vi "UHR-Fleezers Control (host) - 12.6.vi"() -> ()   [LabVIEW 2012] (continued)
            n2300 = Divide(x=w4104, y=w4102) -> (x/y=w4074:dbl[])
            n2301 = Divide(x=w4103, y=w4101) -> (x/y=w4073:dbl[])
            n2302 = Build Array(w4078, w4077, w4108, w4076, w4075, w4105, w4093, w4092, w4074, w4073, w4102, w4101) -> (w4097:dbl[][])
            n2303 = Bundle("T1 Y", "T1 X", "T1 Sum", "T2 Y", "T2 X", "T2 Sum", "T1 FB Sum", "T2 FB Sum", "PSD Y", "PSD X", "PSD Y Sum", "PSD X Sum") -> (w4079:T42)  [unwired: 1 out]
            n2304 = To Word Integer(number=w4112) -> (16bit integer=w4071:i16[])
            n2305 = Cluster To Array(cluster=w4079) -> (array=w4098:string[])
          }
          frame "IR-QPD + PSD + FB-QPD X position" {
            w4184 = 2  # Channel pattern
            # "time average x2 the 3 psd signals (detection laser)"
            # "deinterlace 3 signals from qpds"
            n2306 = Decimate 1D Array(w4204) -> (w4203:i16[], w4202:i16[], w4185:i16[], w4201:i16[], w4147:i16[], w4144:i16[], w4141:i16[], w4172:i16[])
            n2307 = Select(t=i16 -1, s="Flip X Sign", f=i16 1) -> (s? t:f=w4137:i16)
            n2308 = Multiply(x=w4202, y=w4137) -> (x*y=w4138:i16[])
            n2309 = Decimate 1D Array(w4185) -> (w4170:i16[], w4168:i16[])
            n2310 = Decimate 1D Array(w4203) -> (w4200:i16[], w4187:i16[])
            n2311 = Decimate 1D Array(w4138) -> (w4199:i16[], w4197:i16[])
            n2312 = Decimate 1D Array(w4201) -> (w4198:i16[], w4196:i16[])
            n2313 = Decimate 1D Array(w4172) -> (w4171:i16[], w4169:i16[])
            n2314 = call "downsample 1D array - I16.vi"("Ave N"=2.0, "Array In"=w4147) -> ("Array Out"=w4145:i16[])  [unwired: 1 in]
            n2315 = call "downsample 1D array - I16.vi"("Ave N"=2.0, "Array In"=w4141) -> ("Array Out"=w4139:i16[])  [unwired: 1 in]
            n2316 = call "downsample 1D array - I16.vi"("Ave N"=2.0, "Array In"=w4144) -> ("Array Out"=w4142:i16[])  [unwired: 1 in]
            n2317 = Interleave 1D Arrays(w4200, w4199, w4198, w4187, w4197, w4196, w4171, w4170, w4169, w4168, w4145, w4142, w4139) -> (w4195:i16[])
            n2318 = Divide(x=w4195, y=3276.7) -> (x/y=w4194:dbl[])
            n2319 = Decimate 1D Array(w4194) -> (w4193:dbl[], w4192:dbl[], w4191:dbl[], w4190:dbl[], w4189:dbl[], w4188:dbl[], w4160:dbl[], w4158:dbl[], w4157:dbl[], w4155:dbl[], w4154:dbl[], w4153:dbl[], w4150:dbl[])
            n2320 = Negate(x=w4150) -> (-x=w4148:dbl[])
            n2321 = Divide(x=w4154, y=w4150) -> (x/y=w4152:dbl[])
            n2322 = Divide(x=w4153, y=w4148) -> (x/y=w4151:dbl[])
            n2323 = Divide(x=w4193, y=w4191) -> (x/y=w4176:dbl[])
            n2324 = Divide(x=w4192, y=w4191) -> (x/y=w4175:dbl[])
            n2325 = Divide(x=w4190, y=w4188) -> (x/y=w4174:dbl[])
            n2326 = Divide(x=w4189, y=w4188) -> (x/y=w4173:dbl[])
            n2327 = Divide(x=w4160, y=w4158) -> (x/y=w4159:dbl[])
            n2328 = Divide(x=w4157, y=w4155) -> (x/y=w4156:dbl[])
            n2329 = Build Array(w4176, w4175, w4191, w4174, w4173, w4188, w4159, w4158, w4156, w4155, w4152, w4151, w4150) -> (w4149:dbl[][])
            n2330 = Bundle("T1 Y", "T1 X", "T1 Sum", "T2 Y", "T2 X", "T2 Sum", "T1 FB X", "T1 FB Sum", "T2 FB X", "T2 FB Sum", "PSD Y", "PSD X", "PSD Y Sum") -> (w4177:T43)  [unwired: 1 out]
            n2331 = Cluster To Array(cluster=w4177) -> (array=w4186:string[])
          }
          frame "IR-QPD + PSD + FB-QPD XY positions" {
            w4251 = 4  # Channel pattern
            # "time average x2 the 3 psd signals (detection laser)"
            # "deinterlace 3 signals from qpds"
            n2332 = Decimate 1D Array(w4275) -> (w4274:i16[], w4273:i16[], w4252:i16[], w4272:i16[], w4218:i16[], w4264:i16[], w4263:i16[], w4240:i16[])
            n2333 = Decimate 1D Array "Feedback Sum"(w4252) -> (w4236:i16[], w4234:i16[])
            n2334 = Decimate 1D Array "QPD Y"(w4274) -> (w4271:i16[], w4254:i16[])
            n2335 = Decimate 1D Array "QPD X"(w4273) -> (w4270:i16[], w4268:i16[])
            n2336 = Decimate 1D Array "Feedback Y"(w4218) -> (w4217:i16[], w4216:i16[])
            n2337 = Decimate 1D Array "QPD Sum"(w4272) -> (w4269:i16[], w4267:i16[])
            n2338 = Decimate 1D Array "Feedback X"(w4240) -> (w4237:i16[], w4235:i16[])
            n2339 = call "downsample 1D array - double.vi"("Ave N"=2.0, "Array In"=w4264) -> ("Array Out"=w4239:dbl[])  [unwired: 1 out]
            n2340 = call "downsample 1D array - double.vi"("Ave N"=2.0, "Array In"=w4263) -> ("Array Out"=w4238:dbl[])  [unwired: 1 out]
            n2341 = Interleave 1D Arrays(w4271, w4270, w4269, w4254, w4268, w4267, w4217, w4237, w4236, w4216, w4235, w4234, w4239, w4238) -> (w4262:dbl[])
            n2342 = Divide(x=w4262, y=3276.7) -> (x/y=w4261:dbl[])
            n2343 = Decimate 1D Array(w4261) -> (w4260:dbl[], w4259:dbl[], w4258:dbl[], w4257:dbl[], w4256:dbl[], w4255:dbl[], w4213:dbl[], w4227:dbl[], w4211:dbl[], w4212:dbl[], w4225:dbl[], w4209:dbl[], w4223:dbl[], w4221:dbl[])
            n2344 = Negate(x=w4221) -> (-x=w4219:dbl[])
            n2345 = Divide(x=w4223, y=w4219) -> (x/y=w4222:dbl[])
            n2346 = Divide(x=w4212, y=w4209) -> (x/y=w4208:dbl[])
            n2347 = Divide(x=w4213, y=w4211) -> (x/y=w4210:dbl[])
            n2348 = Divide(x=w4260, y=w4258) -> (x/y=w4244:dbl[])
            n2349 = Divide(x=w4259, y=w4258) -> (x/y=w4243:dbl[])
            n2350 = Divide(x=w4257, y=w4255) -> (x/y=w4242:dbl[])
            n2351 = Divide(x=w4256, y=w4255) -> (x/y=w4241:dbl[])
            n2352 = Divide(x=w4227, y=w4211) -> (x/y=w4226:dbl[])
            n2353 = Divide(x=w4225, y=w4209) -> (x/y=w4224:dbl[])
            n2354 = Build Array(w4244, w4243, w4258, w4242, w4241, w4255, w4210, w4226, w4211, w4208, w4224, w4209, w4222, w4221) -> (w4220:dbl[][])
            n2355 = Bundle("T1 Y", "T1 X", "T1 Sum", "T2 Y", "T2 X", "T2 Sum", "T1 FB Y", "T1 FB X", "T1 FB Sum", "T2 FB Y", "T2 FB X", "T2 FB Sum", "PSD X", "PSD Y Sum") -> (w4207:T44)  [unwired: 1 out]
            n2356 = To Word Integer(number=w4262) -> (16bit integer=w4206:i16[])
            n2357 = Cluster To Array(cluster=w4207) -> (array=w4253:string[])
          }
        }
      }
    }
    "AI labels" <- w3282
    n2358 = local read "APD Integration Time (s)"() -> (w3255:dbl)
    n2359 = Array Size(array=w3297) -> (size(s)=w3342:i32)
    n2360 = call <vilib>:"Std Deviation and Variance.vi"("X"=w3244) -> ("standard deviation"=w3243:dbl)  [unwired: 1 in, 2 out]
    n2361 = Add Array Elements(numeric array=w3244) -> (sum=w3245:u32)
    n2362 = Add Array Elements(numeric array=w3297) -> (sum=w3352:u32)
    n2363 = call <vilib>:"Std Deviation and Variance.vi"("X"=w3297) -> ("standard deviation"=w3296:dbl)  [unwired: 1 in, 2 out]
    n2364 = Divide(x=w3243, y=w3085) -> (x/y=w3240:dbl)
    "Rate sigma (Hz) 2" <- w3240
    n2365 = Multiply(x=w3085, y=w3342) -> (x*y=w3087:dbl)
    "Int. Time (s)" <- w3087
    n2366 = Divide(x=w3245, y=w3087) -> (x/y=w3241:dbl)
    "APD 2 Rate (Hz)" <- w3241
    n2367 = Multiply(x="APD Disp. Scale", y=w3248) -> (x*y=w3257:waveform(dbl)[])
    n2368 = Divide(x=w3352, y=w3087) -> (x/y=w3294:dbl)
    "APD 1 Rate (Hz)" <- w3294
    n2369 = Divide(x=w3296, y=w3085) -> (x/y=w3295:dbl)
    "Rate sigma (Hz)" <- w3295
    n2370 = Divide(x=w3240, y=w3241) -> (x/y=→"Sigma/Mean 2":dbl)
    n2371 = Multiply(x="APD Disp. Downsample", y=w3255) -> (x*y=w3253:dbl)
    n2372 = Divide(x=w3295, y=w3294) -> (x/y=→"Sigma/Mean":dbl)
    n2373 = Divide(x=w3257, y=w3253) -> (x/y=w3077:waveform(dbl)[])
    n2374 = Index Array(array=w3077, index=0) -> (element=w3237:waveform(dbl))
    n2375 = Index Array(array=w3077, index=1) -> (element=w3235:waveform(dbl))
    n2376 = Index Array(array=w3077, index=2) -> (element=w3079:waveform(dbl))
    n2377 = Subtract(x=w3237, y="APD 1 Offset") -> (x-y=w3233:waveform(dbl))
    n2378 = Subtract(x=w3235, y="APD 2 Offset") -> (x-y=w3232:waveform(dbl))
    n2379 = Subtract(x=w3079, y="APD 3 Offset") -> (x-y=w3076:waveform(dbl))
    n2380 = Add Array Elements(numeric array=w3086) -> (sum=w3089:u32)
    n2381 = call <vilib>:"Std Deviation and Variance.vi"("X"=w3086) -> ("standard deviation"=w3088:dbl)  [unwired: 1 in, 2 out]
    n2382 = Build Array(w3233, w3232, w3076) -> (→"APD Chart":waveform(dbl)[])
    n2383 = Divide(x=w3089, y=w3087) -> (x/y=w3083:dbl)
    "APD 3 Rate (Hz)" <- w3083
    n2384 = Divide(x=w3088, y=w3085) -> (x/y=w3084:dbl)
    "Rate sigma (Hz) 3" <- w3084
    n2385 = Divide(x=w3084, y=w3083) -> (x/y=→"Sigma/Mean 3":dbl)
    n2386 = local read "Data Period (s)"() -> (w3140:dbl)
    n2387 = local read "BD 1 Frequency 2 (MHz)"() -> (w3173:dbl)
    n2388 = local read "BD 1 Frequency 1 (MHz)"() -> (w3174:dbl)
    n2389 = Decimate 1D Array(w3181) -> (w3205:i16[], w3204:i16[], w3202:i16[], w3201:i16[])  [unwired: 9 out]
    n2390 = Multiply(x=w3140, y="Trap Pos. Disp. Downsample") -> (x*y=w3138:dbl)
    n2391 = Divide(x=w3205, y=w3204) -> (x/y=w3206:dbl[])
    n2392 = Divide(x=w3202, y=w3201) -> (x/y=w3203:dbl[])
    n2393 = local read "AOM X Cal (nm/MHz)"() -> (w3171:dbl)
    n2394 = Split 1D Array(array=w3206, index="N El. to Ave.") -> (second subarray=w3209:dbl[])  [unwired: 1 out]
    n2395 = Split 1D Array(array=w3203, index="N El. to Ave.") -> (second subarray=w3208:dbl[])  [unwired: 1 out]
    n2396 = Multiply(x=w3140, y="Trap Disp. Downsample") -> (x*y=w3219:dbl)
    "Display Period (s)" <- w3219
    n2397 = for "Trap AI" {
      tunnel: [w4000] -> w3384 mode=indexing
      tunnel: w3217 -> [w3991]
      tunnel: "Trap Disp. Downsample" -> [w3998]
      tunnel: w3283 -> [w3996] mode=indexing
      tunnel: w3140 -> [w3995]
      tunnel: w3282 -> [w3994] mode=indexing
      tunnel: [w3993] -> w3252 mode=indexing
      tunnel: w3219 -> [w3992]
      workers-P: _ -> [_]
      n2398 = Bundle By Name("Y"=w3996, "dt"=w3995) -> (w3997:waveform(dbl))  [unwired: 1 out]
      n2399 = Set Waveform Attribute(5:w3994, 6:"NI_ChannelName" ("name"), 7:w3997) -> (3:w3993:waveform(dbl))  [unwired: 1 in, 2 out]
      n2400 = call "downsample 1D array - double.vi"("Ave N"=w3998, "Array In"=w3996) -> ("Array Out"=w3999:dbl[])  [unwired: 1 out]
      n2401 = Bundle By Name(cluster=w3993, "t0"=w3991, "Y"=w3999, "dt"=w3992) -> (w4000:waveform(dbl))
    }
    n2402 = Bundle("BD 1 Frequency 1 (MHz)"=w3174, "BD 1 Frequency 2 (MHz)"=w3173) -> (w3175:T45)  [unwired: 1 out]
    n2403 = call-poly <vilib>:"Mean.vi"("X"=w3208) -> ("mean"=w3196:dbl)  [unwired: 1 out]
    n2404 = call-poly <vilib>:"Mean.vi"("X"=w3209) -> ("mean"=w3197:dbl)  [unwired: 1 out]
    n2405 = Reciprocal(x=w3219) -> (1/x=→"Trap Disp. Freq. (Hz)":dbl)
    n2406 = Cluster To Array(cluster=w3175) -> (array=w3172:dbl[])
    n2407 = local read "Trap X AI1 (DMA)"() -> (w3207:T13)
    n2408 = local read "Data points/scans (MCL)"() -> (w3362:dbl)
    n2409 = To Fixed-Point(number=w3196) -> (fixed-point=w3194:fxp<+/-,16,1>)  [unwired: 1 in]
    n2410 = To Fixed-Point(number=w3197) -> (fixed-point=w3195:fxp<+/-,16,1>)  [unwired: 1 in]
    n2411 = Bundle("Trap 1 Pos.", "Trap 2 Pos.") -> (w3216:cluster{string, string})  [unwired: 1 out]
    n2412 = Bundle By Name(cluster=w3207, "Set 1"=w3195, "Set 2"=w3194) -> (→"Trap X AI1 (DMA)":T13)
    n2413 = Cluster To Array(cluster=w3216) -> (array=w3213:string[])
    n2414 = Unbundle(w3073) -> (w3074:u32[])  [unwired: 2 out]
    n2415 = Select(t=-1.0, s="Negate Y Axis", f=1.0) -> (s? t:f=w3157:dbl)
    n2416 = for "Trap Position" {
      tunnel: w3221 -> [w3592] mode=indexing
      tunnel: "Trap Pos. Disp. Downsample" -> [w3591]
      tunnel: w3138 -> [w3589]
      tunnel: w3217 -> [w3588]
      tunnel: w3213 -> [w3586] mode=indexing
      tunnel: [w3585] -> w3127 mode=indexing
      tunnel: w3172 -> [w3583] mode=indexing
      tunnel: w3171 -> [w3581]
      tunnel: w3157 -> [w3580]
      n2417 = call "downsample 1D array - double.vi"("Ave N"=w3591, "Array In"=w3592) -> ("Array Out"=w3590:dbl[])  [unwired: 1 out]
      n2418 = Subtract(x=w3590, y=w3583) -> (x-y=w3584:dbl[])
      n2419 = Multiply(x=w3581, y=w3584) -> (x*y=w3582:dbl[])
      n2420 = Multiply(x=w3580, y=w3582) -> (x*y=w3579:dbl[])
      n2421 = Bundle By Name("Y"=w3579, "dt"=w3589, "t0"=w3588) -> (w3587:waveform(dbl))  [unwired: 1 out]
      n2422 = Set Waveform Attribute(5:w3586, 6:"NI_ChannelName" ("name"), 7:w3587) -> (3:w3585:waveform(dbl))  [unwired: 1 in, 2 out]
    }
    n2423 = To Double Precision Float(number=w3074) -> (double precision float=w3280:dbl[])
    n2424 = local read "Display Period (s)"() -> (w3269:dbl)
    n2425 = Increment(x=w3362) -> (x+1=w3363:dbl)
    n2426 = Index Array(array=w3127, index=0) -> (element=w3131:waveform(dbl))
    n2427 = Index Array(array=w3127, index=1) -> (element=w3126:waveform(dbl))
    n2428 = feedback #7(w3363) -> (w3366:dbl)
    n2429 = Select(t=0, s=w3353, f=w3366) -> (s? t:f=w3359:dbl)
    n2430 = Array Size(array=w3280) -> (size(s)=w3365:i32)
    n2431 = Build Array (concatenate)(w3248, w3384) -> (w3250:waveform(dbl)[])
    "All Signals" <- w3250
    n2432 = Add(x=w3365, y=w3359) -> (x+y=w3360:dbl)
    n2433 = Unbundle By Name(w3131) -> ("Y"=w3132:dbl[])
    n2434 = Divide(x="Bead Sep. Int. Time (s)", y=w3269) -> (x/y=w3167:dbl)
    n2435 = Add(x=w3132, y="FB Trap Pos Offset") -> (x+y=w3130:dbl[])
    "T1 x pos data" <- w3130
    n2436 = Greater?(x=w3360, y=w3362) -> (0:w3361:bool)
    n2437 = feedback #8(w3130) -> (w3169:dbl[])
    n2438 = Build Array (concatenate)(w3130, w3169) -> (w3168:dbl[])
    n2439 = Bundle By Name(cluster=w3131, "Y"=w3130) -> (w3129:waveform(dbl))
    n2440 = Select(t=w3359, s=w3361, f=w3360) -> (s? t:f=w3358:dbl)
    n2441 = feedback-in #7(w3358) -> ()
    n2442 = local read "MCL Scanning"() -> (w3356:bool)
    n2443 = Bundle(w3129, w3126) -> (w3125:cluster{waveform(dbl), waveform(dbl)})  [unwired: 1 out]
    n2444 = Split 1D Array(array=w3168, index=w3167) -> (first subarray=w3161:dbl[])  [unwired: 1 out]
    n2445 = feedback-in #8(w3161) -> ()
    n2446 = Not(x=w3361) -> (.not. x?=w3355:bool)
    n2447 = Cluster To Array(cluster=w3125) -> (array=w3101:waveform(dbl)[])
    "Trap Positions" <- w3101
    n2448 = call-poly <vilib>:"Mean.vi"("X"=w3161) -> ("mean"=w3160:dbl)  [unwired: 1 out]
    "Mean T1 Position (nm)" <- w3160
    n2449 = Subtract(x=w3161, y=w3160) -> (x-y=w3166:dbl[])
    n2450 = Square(x=w3166) -> (x^2=w3165:dbl[])
    n2451 = And(x=w3355, y=w3356) -> (x .and. y?=w3357:bool)
    n2452 = call-poly <vilib>:"Mean.vi"("X"=w3165) -> ("mean"=w3164:dbl)  [unwired: 1 out]
    n2453 = Square Root(x=w3164) -> (sqrt(x)=w3163:dbl)
    n2454 = Or(x=w3357, y=w3353) -> (x .or. y?=w3354:bool)
    n2455 = Equal?(x="Tab Control 6", y=T35."High Res Display") -> (x = y?=w3286:bool)
    n2456 = Multiply(x=10.0, y=w3163) -> (x*y=→"Trap 1 Position RMS (A)":dbl)
    n2457 = case "For displaying the high resolution display (no downsampling)" shown="True" w3286 {
      tunnel: w3252 -> [_ w3612]
      frame False {
      }
      frame True {
        n2458 = Index Array(array=w3612, index="High Res. Display") -> (element=w3613:waveform(dbl))
        n2459 = call <vilib>:"Std Deviation and Variance.vi"("X"=w3613) -> ("mean"=w3620:dbl, "standard deviation"=w3625:dbl)  [unwired: 1 in, 1 out]
        "Mean Intensity" <- w3620
        "Sigma" <- w3625
        n2460 = Subtract(x=w3613, y=w3620) -> (x-y=w3619:waveform(dbl))
        n2461 = Select(t=w3619, s="Subtract mean", f=w3613) -> (s? t:f=→"1 Channel":waveform(dbl))
        n2462 = Divide(x=w3625, y=w3620) -> (x/y=→"Sigma/Mean":dbl)
        n2463 = feedback #9(1) -> (w3614:i32)
        n2464 = Greater Or Equal?(x=w3614, y="Slow mean N ave.") -> (x >= y?=w3627:bool)
        n2465 = Increment(x=w3614) -> (x+1=w3629:i32)
        n2466 = Select(t=1, s=w3627, f=w3629) -> (s? t:f=w3616:i32)
        n2467 = feedback-in #9(w3616) -> ()
        n2468 = feedback #10() -> (w3617:waveform(dbl))  [unwired: 1 out]
        n2469 = case shown="Default" w3614 {
          tunnel: [w3632 w3635] -> w3618
          tunnel: w3617 -> [w3634 _]
          tunnel: w3613 -> [w3633 w3635]
          frame Default {
            n2470 = call-poly <vilib>:"Append Waveforms.vi"("waveform B"=w3633, "waveform A"=w3634) -> ("waveform out"=w3632:waveform(dbl))  [unwired: 1 in, 8 out]
          }
          frame 1 {
          }
        }
        n2471 = feedback-in #10(w3618) -> ()
        n2472 = case shown="True" w3627 {
          tunnel: w3618 -> [_ w3631]
          frame False {
          }
          frame True {
            n2473 = call-poly <vilib>:"Mean.vi"("X"=w3631) -> ("mean"=→"Slow mean":dbl)  [unwired: 1 out]
          }
        }
      }
    }
    n2474 = case "For plotting results of scanning MCL (fluorescence and detection laser images)" shown="True" w3354 {
      tunnel: w3353 -> [_ w3739]
      tunnel: w3362 -> [_ _]
      tunnel: w3252 -> [_ w3868]
      tunnel: w3230 -> [_ w3776]
      tunnel: w3073 -> [_ w3746]
      frame False {
      }
      frame True {
        w3756 = u32 0 items=["Horizontal", "Vertical", "Central", "1st Diagonal", "2nd Diagonal"] ("Type of Symmetry")
        w3783 = u32 0 items=["Horizontal", "Vertical", "Central", "1st Diagonal", "2nd Diagonal"] ("Type of Symmetry")
        w3807 = u32 0 items=["Horizontal", "Vertical", "Central", "1st Diagonal", "2nd Diagonal"] ("Type of Symmetry")
        w3810 = u32 0 items=["Horizontal", "Vertical", "Central", "1st Diagonal", "2nd Diagonal"] ("Type of Symmetry")
        w3839 = u32 0 items=["Horizontal", "Vertical", "Central", "1st Diagonal", "2nd Diagonal"] ("Type of Symmetry")
        n2475 = Unbundle(w3746) -> (w3745:u32[], w3743:u32[], w3741:u32[])
        n2476 = To Double Precision Float(number=w3745) -> (double precision float=w3744:dbl[])
        n2477 = To Double Precision Float(number=w3743) -> (double precision float=w3742:dbl[])
        n2478 = To Double Precision Float(number=w3741) -> (double precision float=w3740:dbl[])
        n2479 = Index Array(array=w3868, index=10) -> (element=w3874:waveform(dbl))
        n2480 = Index Array(array=w3868, index=11) -> (element=w3871:waveform(dbl))
        n2481 = local read "Cycles/step (MCL)"() -> (w3824:u64)
        n2482 = Index Array(array=w3868, index="Channel") -> (element=w3870:waveform(dbl))
        n2483 = Unbundle(w3776) -> ("New Image"=w3775:T2, "New Image"=w3774:T2, "New Image"=w3747:T2, "New Image"=w3748:T2, "New Image"=w3749:T2)
        n2484 = local read "Scan steps (MCL)"() -> (w3735:u64)
        n2485 = Unbundle By Name(w3874) -> ("Y"=w3826:dbl[])
        n2486 = Unbundle By Name(w3871) -> ("Y"=w3828:dbl[])
        n2487 = local read "Scan lines (y)"() -> (w3736:u64)
        n2488 = local read "N APD Samp/step"() -> (w3738:dbl)
        n2489 = Unbundle By Name(w3870) -> ("Y"=w3833:dbl[])
        n2490 = call "downsample 1D array - double.vi"("Ave N"=w3824, "Array In"=w3826) -> ("Array Out"=w3825:dbl[])  [unwired: 1 out]
        n2491 = call "downsample 1D array - double.vi"("Ave N"=w3824, "Array In"=w3828) -> ("Array Out"=w3827:dbl[])  [unwired: 1 out]
        n2492 = call "downsample 1D array - double.vi"("Ave N"=w3824, "Array In"=w3833) -> ("Array Out"=w3832:dbl[])  [unwired: 1 out]
        n2493 = Multiply(x=w3735, y=u64 2) -> (x*y=w3737:u64)
        n2494 = feedback #11(w3742) -> (w3801:dbl[])
        n2495 = Build Array (concatenate)(w3801, w3742) -> (w3800:dbl[])
        n2496 = feedback #12(w3740) -> (w3773:dbl[])
        n2497 = Build Array (concatenate)(w3773, w3740) -> (w3734:dbl[])
        n2498 = Select(t=w3742, s=w3739, f=w3800) -> (s? t:f=w3785:dbl[])
        n2499 = feedback-in #11(w3785) -> ()
        n2500 = Select(t=w3740, s=w3739, f=w3734) -> (s? t:f=w3758:dbl[])
        n2501 = feedback-in #12(w3758) -> ()
        n2502 = feedback #13(w3744) -> (w3894:dbl[])
        n2503 = Build Array (concatenate)(w3894, w3744) -> (w3876:dbl[])
        n2504 = Select(t=w3744, s=w3739, f=w3876) -> (s? t:f=w3880:dbl[])
        n2505 = feedback-in #13(w3880) -> ()
        n2506 = feedback #14(w3825) -> (w3882:dbl[])
        n2507 = Build Array (concatenate)(w3882, w3825) -> (w3873:dbl[])
        n2508 = feedback #15(w3832) -> (w3892:dbl[])
        n2509 = Build Array (concatenate)(w3892, w3832) -> (w3891:dbl[])
        n2510 = feedback #16(w3827) -> (w3884:dbl[])
        n2511 = Build Array (concatenate)(w3884, w3827) -> (w3885:dbl[])
        n2512 = Select(t=w3825, s=w3739, f=w3873) -> (s? t:f=w3829:dbl[])
        n2513 = feedback-in #14(w3829) -> ()
        n2514 = Select(t=w3832, s=w3739, f=w3891) -> (s? t:f=w3831:dbl[])
        n2515 = feedback-in #15(w3831) -> ()
        n2516 = Select(t=w3827, s=w3739, f=w3885) -> (s? t:f=w3830:dbl[])
        n2517 = feedback-in #16(w3830) -> ()
        n2518 = call "integrate 1D array interval - double.vi"("Ave N"=w3738, "Array In"=w3785) -> ("Array Out"=w3796:dbl[])  [unwired: 1 out]
        n2519 = call "integrate 1D array interval - double.vi"("Ave N"=w3738, "Array In"=w3758) -> ("Array Out"=w3769:dbl[])  [unwired: 1 out]
        n2520 = call "integrate 1D array interval - double.vi"("Ave N"=w3738, "Array In"=w3880) -> ("Array Out"=w3879:dbl[])  [unwired: 1 out]
        n2521 = Array Size(array=w3796) -> (size(s)=w3797:i32)
        n2522 = Array Size(array=w3769) -> (size(s)=w3770:i32)
        n2523 = Array Size(array=w3879) -> (size(s)=w3881:i32)
        n2524 = Multiply(x=w3736, y=w3737) -> (x*y=w3799:u64)
        n2525 = Multiply(x=w3736, y=w3737) -> (x*y=w3772:u64)
        n2526 = Multiply(x=w3736, y=w3737) -> (x*y=w3889:u64)
        n2527 = Subtract(x=w3799, y=w3797) -> (x-y=w3790:u64)
        n2528 = call-poly <vilib>:"Mean.vi"("X"=w3796) -> ("mean"=w3787:dbl)  [unwired: 1 out]
        n2529 = Subtract(x=w3772, y=w3770) -> (x-y=w3763:u64)
        n2530 = call-poly <vilib>:"Mean.vi"("X"=w3769) -> ("mean"=w3760:dbl)  [unwired: 1 out]
        n2531 = Subtract(x=w3889, y=w3881) -> (x-y=w3823:u64)
        n2532 = call-poly <vilib>:"Mean.vi"("X"=w3879) -> ("mean"=w3820:dbl)  [unwired: 1 out]
        n2533 = call-poly <vilib>:"Mean.vi"("X"=w3829) -> ("mean"=w3813:dbl)  [unwired: 1 out]
        n2534 = call-poly <vilib>:"Mean.vi"("X"=w3831) -> ("mean"=w3818:dbl)  [unwired: 1 out]
        n2535 = call-poly <vilib>:"Mean.vi"("X"=w3830) -> ("mean"=w3816:dbl)  [unwired: 1 out]
        n2536 = Initialize Array(1.0 ("element"), w3790) -> (w3786:dbl[])
        n2537 = Initialize Array(1.0 ("element"), w3763) -> (w3759:dbl[])
        n2538 = Initialize Array(1.0 ("element"), w3823) -> (w3814:dbl[])
        n2539 = Multiply(x=w3786, y=w3787) -> (x*y=w3788:dbl[])
        n2540 = Multiply(x=w3759, y=w3760) -> (x*y=w3761:dbl[])
        n2541 = Multiply(x=w3814, y=w3820) -> (x*y=w3821:dbl[])
        n2542 = Multiply(x=w3814, y=w3816) -> (x*y=w3817:dbl[])
        n2543 = Multiply(x=w3814, y=w3818) -> (x*y=w3819:dbl[])
        n2544 = Multiply(x=w3814, y=w3813) -> (x*y=w3815:dbl[])
        n2545 = Build Array (concatenate)(w3796, w3788) -> (w3798:dbl[])
        n2546 = Build Array (concatenate)(w3769, w3761) -> (w3771:dbl[])
        n2547 = Build Array (concatenate)(w3879, w3821) -> (w3888:dbl[])
        n2548 = Build Array (concatenate)(w3829, w3815) -> (w3883:dbl[])
        n2549 = Build Array (concatenate)(w3831, w3819) -> (w3887:dbl[])
        n2550 = Build Array (concatenate)(w3830, w3817) -> (w3886:dbl[])
        n2551 = Reshape Array(w3798, w3736, w3737) -> (w3794:dbl[][])
        n2552 = Reshape Array(w3771, w3736, w3737) -> (w3767:dbl[][])
        n2553 = Reshape Array(w3888, w3736, w3737) -> (w3866:dbl[][])
        n2554 = Reshape Array(w3883, w3736, w3737) -> (w3849:dbl[][])
        n2555 = Reshape Array(w3887, w3736, w3737) -> (w3841:dbl[][])
        n2556 = Reshape Array(w3886, w3736, w3737) -> (w3856:dbl[][])
        n2557 = Array Subset(array=w3794, index (col)=0 ("index"), length (col)=w3735) -> (w3793:dbl[][])  [unwired: 2 in]
        n2558 = Array Subset(array=w3794, index (col)=w3735) -> (w3791:dbl[][])  [unwired: 3 in]
        n2559 = Array Subset(array=w3767, index (col)=0 ("index"), length (col)=w3735) -> (w3766:dbl[][])  [unwired: 2 in]
        n2560 = Array Subset(array=w3767, index (col)=w3735) -> (w3764:dbl[][])  [unwired: 3 in]
        n2561 = Array Subset(array=w3856, index (col)=0 ("index"), length (col)=w3735) -> (w3861:dbl[][])  [unwired: 2 in]
        n2562 = Array Subset(array=w3856, index (col)=w3735) -> (w3859:dbl[][])  [unwired: 3 in]
        n2563 = Array Subset(array=w3866, index (col)=0 ("index"), length (col)=w3735) -> (w3865:dbl[][])  [unwired: 2 in]
        n2564 = Array Subset(array=w3866, index (col)=w3735) -> (w3863:dbl[][])  [unwired: 3 in]
        n2565 = Array Subset(array=w3841, index (col)=0 ("index"), length (col)=w3735) -> (w3847:dbl[][])  [unwired: 2 in]
        n2566 = Array Subset(array=w3841, index (col)=w3735) -> (w3845:dbl[][])  [unwired: 3 in]
        n2567 = Array Subset(array=w3849, index (col)=0 ("index"), length (col)=w3735) -> (w3854:dbl[][])  [unwired: 2 in]
        n2568 = Array Subset(array=w3849, index (col)=w3735) -> (w3852:dbl[][])  [unwired: 3 in]
        n2569 = for {
          tunnel: w3793 -> [w3898] mode=indexing
          tunnel: [w3897] -> w3792 mode=indexing
          workers-P: _ -> [_]
          n2570 = Reverse 1D Array(array=w3898) -> (reversed array=w3897:dbl[])
        }
        n2571 = for {
          tunnel: w3766 -> [w3896] mode=indexing
          tunnel: [w3895] -> w3765 mode=indexing
          workers-P: _ -> [_]
          n2572 = Reverse 1D Array(array=w3896) -> (reversed array=w3895:dbl[])
        }
        n2573 = for {
          tunnel: w3861 -> [w3904] mode=indexing
          tunnel: [w3903] -> w3860 mode=indexing
          workers-P: _ -> [_]
          n2574 = Reverse 1D Array(array=w3904) -> (reversed array=w3903:dbl[])
        }
        n2575 = for {
          tunnel: w3865 -> [w3906] mode=indexing
          tunnel: [w3905] -> w3864 mode=indexing
          workers-P: _ -> [_]
          n2576 = Reverse 1D Array(array=w3906) -> (reversed array=w3905:dbl[])
        }
        n2577 = for {
          tunnel: w3847 -> [w3900] mode=indexing
          tunnel: [w3899] -> w3846 mode=indexing
          workers-P: _ -> [_]
          n2578 = Reverse 1D Array(array=w3900) -> (reversed array=w3899:dbl[])
        }
        n2579 = for {
          tunnel: w3854 -> [w3902] mode=indexing
          tunnel: [w3901] -> w3853 mode=indexing
          workers-P: _ -> [_]
          n2580 = Reverse 1D Array(array=w3902) -> (reversed array=w3901:dbl[])
        }
        n2581 = Index Array(array=w3866, index (row)=0) -> (element=→"Waveform Graph":dbl[])  [unwired: 1 in]
        n2582 = Add(x=w3792, y=w3791) -> (x+y=w3778:dbl[][])
        n2583 = Add(x=w3765, y=w3764) -> (x+y=w3751:dbl[][])
        n2584 = Add(x=w3860, y=w3859) -> (x+y=w3858:dbl[][])
        n2585 = Add(x=w3864, y=w3863) -> (x+y=w3838:dbl[][])
        n2586 = Add(x=w3846, y=w3845) -> (x+y=w3844:dbl[][])
        n2587 = Add(x=w3853, y=w3852) -> (x+y=w3851:dbl[][])
        n2588 = Divide(x=w3844, y=2) -> (x/y=w3842:dbl[][])
        n2589 = Divide(x=w3858, y=2) -> (x/y=w3803:dbl[][])
        n2590 = To Single Precision Float(number=w3838) -> (single precision float=w3837:sgl[][])
        n2591 = To Single Precision Float(number=w3778) -> (single precision float=w3782:sgl[][])
        n2592 = To Single Precision Float(number=w3751) -> (single precision float=w3755:sgl[][])
        n2593 = Divide(x=w3851, y=2) -> (x/y=w3805:dbl[][])
        n2594 = Transpose 2D Array(2D array=w3842) -> (transposed array=→"Data map":dbl[][])
        n2595 = To Single Precision Float(number=w3803) -> (single precision float=w3809:sgl[][])
        n2596 = To Single Precision Float(number=w3805) -> (single precision float=w3806:sgl[][])
        n2597 = call "IMAQ ArrayToImage"("Image Pixels (Float)"=w3837, "Image"=w3775) -> ("Image Out"=w3840:T2)  [unwired: 8 in, 1 out]
        n2598 = call "IMAQ ArrayToImage"("Image Pixels (Float)"=w3782, "Image"=w3774) -> ("Image Out"=w3784:T2)  [unwired: 8 in, 1 out]
        n2599 = call "IMAQ ArrayToImage"("Image Pixels (Float)"=w3755, "Image"=w3747) -> ("Image Out"=w3757:T2)  [unwired: 8 in, 1 out]
        n2600 = call "IMAQ ArrayToImage"("Image Pixels (Float)"=w3809, "Image"=w3748) -> ("Image Out"=w3811:T2)  [unwired: 8 in, 1 out]
        n2601 = call "IMAQ Symmetry"("Type of Symmetry"=w3839, "Image Src"=w3840) -> ("Image Dst Out"=w3835:T2)  [unwired: 3 in, 1 out]
        n2602 = call "IMAQ ArrayToImage"("Image Pixels (Float)"=w3806, "Image"=w3749) -> ("Image Out"=w3808:T2)  [unwired: 8 in, 1 out]
        n2603 = call "IMAQ Symmetry"("Type of Symmetry"=w3783, "Image Src"=w3784) -> ("Image Dst Out"=w3780:T2)  [unwired: 3 in, 1 out]
        n2604 = call "IMAQ Symmetry"("Type of Symmetry"=w3756, "Image Src"=w3757) -> ("Image Dst Out"=w3753:T2)  [unwired: 3 in, 1 out]
        n2605 = call "IMAQ Symmetry"("Type of Symmetry"=w3810, "Image Src"=w3811) -> ("Image Dst Out"=→"Detection Laser X":T2)  [unwired: 3 in, 1 out]
        n2606 = call "IMAQ Symmetry"("Type of Symmetry"=w3807, "Image Src"=w3808) -> ("Image Dst Out"=→"Detection Laser Y":T2)  [unwired: 3 in, 1 out]
        n2607 = call "IMAQ Set Simple Calibration"("Calibration Axis Info"=T36 {"Origin Pixel"={"X"=0.0, "Y"=0.0}, "Angle Relative to Horizontal (deg)"=0.0, "Axis Reference"=0}, "Grid Descriptor"=T37 {"X Step"=0.3, "Y Step"=0.3, "Unit"=enum."Undefined"}, "Image"=w3835) -> ("Calibrated Image"=→"APD 1":T2)  [unwired: 7 in, 1 out]
        n2608 = call "IMAQ Set Simple Calibration"("Calibration Axis Info"=T36 {"Origin Pixel"={"X"=0.0, "Y"=0.0}, "Angle Relative to Horizontal (deg)"=0.0, "Axis Reference"=0}, "Grid Descriptor"=T37 {"X Step"=0.3, "Y Step"=0.3, "Unit"=enum."Undefined"}, "Image"=w3780) -> ("Calibrated Image"=→"APD 2":T2)  [unwired: 7 in, 1 out]
        n2609 = call "IMAQ Set Simple Calibration"("Calibration Axis Info"=T36 {"Origin Pixel"={"X"=0.0, "Y"=0.0}, "Angle Relative to Horizontal (deg)"=0.0, "Axis Reference"=0}, "Grid Descriptor"=T37 {"X Step"=0.3, "Y Step"=0.3, "Unit"=enum."Undefined"}, "Image"=w3753) -> ("Calibrated Image"=→"APD 3":T2)  [unwired: 7 in, 1 out]
      }
    }
    n2610 = case "For computing FFTs for display" shown="True" "Compute FFT" {
      tunnel: w3252 -> [_ w4378]
      frame False {
      }
      frame True {
        n2611 = Build Array("FFT 1 Choice 1", "FFT 1 Choice 2", "FFT 2 Choice 1", "FFT 2 Choice 2") -> (w4371:u16[])
        n2612 = Array Size(array=w4378) -> (size(s)=w4377:i32)
        n2613 = feedback-in #17(w4371) -> ()
        n2614 = feedback #17(u16[] [100, 100, 100, 100]) -> (w4372:u16[])
        n2615 = feedback-in #18("# Spectra to Ave.") -> ()
        n2616 = feedback #18("# Spectra to Ave.") -> (w4369:dbl)
        n2617 = Not Equal?(x="# Spectra to Ave.", y=w4369) -> (x != y?=w4368:bool)
        n2618 = Not Equal?(x=w4371, y=w4372) -> (x != y?=w4370:bool)
        n2619 = feedback #19(1.0) -> (w4355:dbl)
        n2620 = Compound Arithmetic op=OR("Reset FFT", w4370, w4368) -> (w4353:bool)
        n2621 = Select(t=1.0, s=w4353, f=w4355) -> (s? t:f=w4357:dbl)
        n2622 = Greater?(x=w4357, y="# Spectra to Ave.") -> (0:w4376:bool)
        n2623 = Increment(x=w4357) -> (x+1=w4356:dbl)
        n2624 = feedback-in #19(w4356) -> ()
        n2625 = local read "DMA Update Period (s)"() -> (w4351:dbl)
        n2626 = Multiply(x="# Spectra to Ave.", y=w4351) -> (x*y=→"Ave. Time (s)":dbl)
        n2627 = Build Array(cluster{"f0":dbl, "df":dbl, "magnitude":dbl[]} {"f0"=0.0, "df"=0.0, "magnitude"=[]} ("PSD")) -> (w4360:cluster{"f0":dbl, "df":dbl, "magnitude":dbl[]}[])
        n2628 = Build Array(w4360, w4360, w4360, w4360) -> (w4362:T46)
        n2629 = feedback #20(w4362) -> (w4367:T46)
        n2630 = for {
          N: 4 -> [_]
          tunnel: w4371 -> [w4400] mode=indexing
          tunnel: w4378 -> [w4401]
          tunnel: w4377 -> [w4403]
          tunnel: w4353 -> [w4396]
          tunnel: w4376 -> [w4395]
          tunnel: "# Spectra to Ave." -> [w4394]
          tunnel: [w4393] -> w4366 mode=indexing
          tunnel: w4367 -> [w4398] mode=indexing
          tunnel: [w4397] -> w4354 mode=indexing
          tunnel: w4357 -> [w4392]
          n2631 = Less?(x=w4400, y=w4403) -> (x < y?=w4402:bool)
          n2632 = Index Array(array=w4401, index=w4400) -> (element=w4399:waveform(dbl))
          n2633 = case shown="True" w4402 {
            tunnel: w4399 -> [_ w4420]
            tunnel: w4398 -> [w4405 w4418]
            tunnel: [w4405 w4406] -> w4397
            tunnel: w4396 -> [_ w4417]
            tunnel: w4395 -> [_ w4410]
            tunnel: w4394 -> [_ w4409]
            tunnel: [cluster{"f0":dbl, "df":dbl, "magnitude":dbl[]} {"f0"=0.0, "df"=0.0, "magnitude"=[]} ("PSD") w4411] -> w4393
            tunnel: w4392 -> [_ w4408]
            frame False {
            }
            frame True {
              n2634 = call <vilib>:"Std Deviation and Variance.vi"("X"=w4420) -> ("mean"=w4421:dbl)  [unwired: 1 in, 2 out]
              n2635 = Subtract(x=w4420, y=w4421) -> (x-y=w4419:waveform(dbl))
              n2636 = xnode "Spectral Measurements"("Signals"=w4419) -> ("PSD"=w4413:cluster{"f0":dbl, "df":dbl, "magnitude":dbl[]})  [unwired: 1 in, 1 out]
              n2637 = case shown="False" w4417 {
                tunnel: w4418 -> [w4430 _]
                tunnel: [w4426 w4435] -> w4406
                tunnel: w4413 -> [w4429 w4436]
                tunnel: w4410 -> [w4428 _]
                frame False {
                  n2638 = Build Array (concatenate)(w4430, w4429) -> (w4427:cluster{"f0":dbl, "df":dbl, "magnitude":dbl[]}[])
                  n2639 = case shown="True" w4428 {
                    tunnel: w4427 -> [w4431 w4434]
                    tunnel: [w4431 w4432] -> w4426
                    frame False {
                    }
                    frame True {
                      n2640 = Delete From Array(array=w4434, index=0) -> (array with subset deleted=w4432:cluster{"f0":dbl, "df":dbl, "magnitude":dbl[]}[])  [unwired: 1 in, 1 out]
                    }
                  }
                }
                frame True {
                  n2641 = Build Array(w4436) -> (w4435:cluster{"f0":dbl, "df":dbl, "magnitude":dbl[]}[])
                }
              }
              n2642 = for {
                tunnel: w4406 -> [w4425] mode=indexing
                tunnel: [w4424] -> w4416 mode=indexing
                workers-P: _ -> [_]
                n2643 = Unbundle By Name(w4425) -> ("magnitude"=w4424:dbl[])
              }
              n2644 = Transpose 2D Array(2D array=w4416) -> (transposed array=w4415:dbl[][])
              n2645 = for {
                tunnel: w4415 -> [w4423] mode=indexing
                tunnel: [w4422] -> w4414 mode=indexing
                workers-P: _ -> [_]
                n2646 = Add Array Elements(numeric array=w4423) -> (sum=w4422:dbl)
              }
              n2647 = Select(t=w4409, s=w4410, f=w4408) -> (s? t:f=w4407:dbl)
              n2648 = Divide(x=w4414, y=w4407) -> (x/y=w4412:dbl[])
              n2649 = Bundle By Name(cluster=w4413, "magnitude"=w4412) -> (w4411:cluster{"f0":dbl, "df":dbl, "magnitude":dbl[]})
            }
          }
        }
        n2650 = case shown="True" w4353 {
          tunnel: w4354 -> [w4385 w4391]
          tunnel: [w4385 w4386] -> w4352
          frame False {
          }
          frame True {
            n2651 = Array Subset(array=w4391, index (row)=0 ("index"), length (row)=4 ("length"), index (col)=0 ("index"), length (col)=1 ("length")) -> (w4386:T46)
          }
        }
        n2652 = feedback-in #20(w4352) -> ()
        n2653 = Split 1D Array(array=w4366, index=2) -> (first subarray=→"FFT 1":cluster{"f0":dbl, "df":dbl, "magnitude":dbl[]}[], second subarray=→"FFT 2":cluster{"f0":dbl, "df":dbl, "magnitude":dbl[]}[])
      }
    }
    n2654 = Index Array(array=w3250, index=4) -> (element=w3306:waveform(dbl))
    n2655 = Index Array(array=w3250, index=7) -> (element=w3303:waveform(dbl))
    n2656 = Divide(x="T1 offset_x (mV)", y=1000.0) -> (x/y=w3307:dbl)
    n2657 = feedback-in #21("Calibration") -> ()
    n2658 = feedback #21(u16 1 ("Calibration")) -> (w3325:u16)
    n2659 = Divide(x="T2 offset_x (mV)", y=1000.0) -> (x/y=w3305:dbl)
    n2660 = case shown="2" "Calibration" {
      tunnel: "T1 alpha_x (nm/V)" -> [_ w3699 w3720]
      tunnel: "T1 kappa_x (pN/nm)" -> [_ _ w3710]
      tunnel: "T2 alpha_x (nm/V)" -> [_ w3698 w3718]
      tunnel: "T2 kappa_x (pN/nm)" -> [_ _ w3711]
      tunnel: w3306 -> [w3681 w3696 w3716]
      tunnel: w3303 -> [w3680 w3694 w3714]
      tunnel: [w3681 w3693 w3713] -> w3334
      tunnel: [w3680 w3692 w3712] -> w3333
      tunnel: ["T1 X (V)" ("Label.Text") "T1 X (nm)" ("Label.Text") "T1 X (pN)" ("Label.Text")] -> w3322
      tunnel: ["T2 X (V)" ("Label.Text") "T2 X (nm)" ("Label.Text") "T2 X (pN)" ("Label.Text")] -> w3321
      tunnel: ["Position (V)" ("Label.Text") "Position (nm)" ("Label.Text") "Force (pN)" ("Label.Text")] -> w3323
      tunnel: w3305 -> [_ w3684 w3703]
      tunnel: w3307 -> [_ w3687 w3705]
      tunnel: ["Mean (V)" ("Label.Text") "Mean (nm)" ("Label.Text") "Mean (pN)" ("Label.Text")] -> w3318
      tunnel: ["Difference (V)" ("Label.Text") "Difference (nm)" ("Label.Text") "Difference (pN)" ("Label.Text")] -> w3258
      frame 0, Default {
      }
      frame 1 {
        n2661 = Unbundle By Name(w3696) -> ("Y"=w3700:dbl[])
        n2662 = Unbundle By Name(w3694) -> ("Y"=w3685:dbl[])
        n2663 = Subtract(x=w3700, y=w3687) -> (x-y=w3688:dbl[])
        n2664 = Subtract(x=w3685, y=w3684) -> (x-y=w3686:dbl[])
        n2665 = Multiply(x=w3686, y=w3698) -> (x*y=w3695:dbl[])
        n2666 = Multiply(x=w3699, y=w3688) -> (x*y=w3697:dbl[])
        n2667 = Bundle By Name(cluster=w3694, "Y"=w3695) -> (w3692:waveform(dbl))
        n2668 = Bundle By Name(cluster=w3696, "Y"=w3697) -> (w3693:waveform(dbl))
      }
      frame 2 {
        n2669 = Unbundle By Name(w3716) -> ("Y"=w3721:dbl[])
        n2670 = Unbundle By Name(w3714) -> ("Y"=w3719:dbl[])
        n2671 = Subtract(x=w3719, y=w3703) -> (x-y=w3704:dbl[])
        n2672 = Subtract(x=w3721, y=w3705) -> (x-y=w3706:dbl[])
        n2673 = Compound Arithmetic op=MULTIPLY(w3704, w3718, w3711) -> (w3715:dbl[])
        n2674 = Compound Arithmetic op=MULTIPLY(w3710, w3720, w3706) -> (w3717:dbl[])
        n2675 = Bundle By Name(cluster=w3714, "Y"=w3715) -> (w3712:waveform(dbl))
        n2676 = Bundle By Name(cluster=w3716, "Y"=w3717) -> (w3713:waveform(dbl))
      }
    }
    n2677 = case shown="True" "Read Lateness and Rel Phase" {
      tunnel: w3124 -> [w3636 w3669]
      tunnel: w3123 -> [w3637 w3668]
      tunnel: [w3636 w3641] -> w3300
      tunnel: [w3637 w3640] -> w3299
      frame False {
      }
      frame True {
        n2678 = xnode "Read/Write Control"("FPGA VI Reference In"=w3669, "error in"=w3668) -> ("FPGA VI Reference Out"=w3643:T20, "error out"=w3642:errorcluster, "GI Relative phase"=→"GI relative phase":i16, "Relative phase"=→"Relative phase (AI1)":i16, "AI Late Counter"=→"Late Counter (AI1)":u8, "GI Late Counter"=→"GI Late Counter":u8, "MCL Late Counter"=→"MCL Late Counter":u8, "MCL Relative Phase"=→"Relative Phase (MCL)":i16, "APD Acq Relative Phase"=→"APD Acq Relative Phase":i16, "APD 1 Gate Relative Phase"=→"APD 1 Gate Relative Phase":i16, "APD 2 Gate Relative Phase"=→"APD 2 Gate Relative Phase":i16, "APD Acq Late Counter"=→"APD Acq Late Counter":u8, "APD 1 Gate Late Counter"=→"APD 1 Gate Late Counter":u8, "APD 2 Gate Late Counter"=→"APD 2 Gate Late Counter":u8, "Green FB Relative Phase"=→"Relative phase (Green FB)":i16, "GI Relative phase 2"=→"GI relative phase 2":i16, "GI Late Counter 2"=→"GI Late Counter 2":u8, "Trap Pos FIFO Timeout"=→"Trap Pos FIFO Timeout":u16, "Trap AI FIFO Timeout"=→"Trap AI FIFO Timeout":u16, "RI Late Counter"=→"RI Late Counter":u8, "RI Relative phase"=→"RI relative phase":i16, "Green Late Counter"=→"Green AI Late Counter":u8, "BI Late Counter (AO)"=→"Late Counter (BI AO)":u8, "Blue Late Counter (D)"=→"Late Counter (BI DO)":u8, "BI Relative phase (AO)"=→"Relative phase (BI AO)":i16, "BI Relative phase (D)"=→"Relative phase (BI DO)":i16)
        n2679 = xnode "Read/Write Control"("FPGA VI Reference In"=w3643, "error in"=w3642) -> ("FPGA VI Reference Out"=w3641:T20, "error out"=w3640:errorcluster, "APD 3 Gate Late Counter"=→"APD 3 Gate Late Counter":u8, "APD 3 Gate Relative Phase"=→"APD 3 Gate Relative Phase":i16)
      }
    }
    n2680 = Not Equal?(x=w3325, y="Calibration") -> (x != y?=w3284:bool)
    n2681 = case shown="True" w3284 {
      tunnel: w3323 -> [_ w3674]
      tunnel: w3322 -> [_ w3673]
      tunnel: w3321 -> [_ w3672]
      tunnel: w3318 -> [_ w3671]
      tunnel: w3258 -> [_ w3670]
      frame False {
      }
      frame True {
        n2682 = property on="Force" class="WFChart (strict)"("YScale.NameLbl.Text"=w3674) -> ()  [unwired: 2 in, 2 out]
        n2683 = property on="T2 X" class="DigNum (strict)"("Caption.Text"=w3672) -> ()  [unwired: 2 in, 2 out]
        n2684 = property on="T1 X" class="DigNum (strict)"("Caption.Text"=w3673) -> ()  [unwired: 2 in, 2 out]
        n2685 = property on="Mean" class="DigNum (strict)"("Caption.Text"=w3671) -> ()  [unwired: 2 in, 2 out]
        n2686 = property on="Difference" class="DigNum (strict)"("Caption.Text"=w3670) -> ()  [unwired: 2 in, 2 out]
      }
    }
    n2687 = Unbundle By Name(w3306) -> ("Y"=w3309:dbl[])
    n2688 = Unbundle By Name(w3303) -> ("Y"=w3312:dbl[])
    n2689 = Subtract(x=w3309, y=w3307) -> (x-y=w3310:dbl[])
    n2690 = Subtract(x=w3312, y=w3305) -> (x-y=w3311:dbl[])
    n2691 = Multiply(x=w3311, y="T2 alpha_x (nm/V)") -> (x*y=w3106:dbl[])
    n2692 = Multiply(x="T1 alpha_x (nm/V)", y=w3310) -> (x*y=w3107:dbl[])
    n2693 = Not(x="Trap Trig. Fl.") -> (.not. x?=w3143:bool)
    n2694 = Multiply(x=w3333, y=-1.0) -> (x*y=w3314:waveform(dbl))
    n2695 = Subtract(x=w3107, y=w3106) -> (x-y=w3302:dbl[])
    n2696 = Unbundle By Name(w3333) -> ("Y"=w3274:dbl[])
    n2697 = Unbundle By Name(w3334) -> ("Y"=w3108:dbl[])
    n2698 = Negate(x=w3302) -> (-x=w3104:dbl[])
    n2699 = Build Array(w3334, w3314) -> (→"Force":waveform(dbl)[])
    n2700 = Subtract(x=w3104, y="Offset (nm)") -> (x-y=w3272:dbl[])
    n2701 = call-poly <vilib>:"Mean.vi"("X"=w3274) -> ("mean"=w3110:dbl)  [unwired: 1 out]
    "T2 X" <- w3110
    n2702 = Negate(x=w3274) -> (-x=w3275:dbl[])
    n2703 = call-poly <vilib>:"Mean.vi"("X"=w3108) -> ("mean"=w3111:dbl)  [unwired: 1 out]
    "T1 X" <- w3111
    n2704 = Negate(x=w3110) -> (-x=w3109:dbl)
    n2705 = Bundle By Name(cluster=w3306, "Y"=w3272) -> (w3249:waveform(dbl))
    "Bead Separation" <- w3249
    n2706 = Add(x=w3108, y=w3275) -> (x+y=w3276:dbl[])
    n2707 = Add(x=w3111, y=w3109) -> (x+y=w3320:dbl)
    n2708 = Subtract(x=w3111, y=w3109) -> (x-y=→"Difference":dbl)
    n2709 = Divide(x=w3276, y=2.0) -> (x/y=→"Vec Mean of T1 T2":dbl[])
    n2710 = Divide(x=w3320, y=2.0) -> (x/y=w3278:dbl)
    "Mean" <- w3278
    n2711 = feedback-in #22("Trap Trig. Fl.") -> ()
    n2712 = feedback #22("Trap Trig. Fl.") -> (w3141:bool)
    n2713 = And(x=w3143, y=w3141) -> (x .and. y?=w3142:bool)
    n2714 = case "If have just turned off triggering" shown="True" w3142 {
      tunnel: w3124 -> [_ w3471]
      tunnel: w3123 -> [_ w3470]
      frame False {
      }
      frame True {
        w3469 = FALSE ("FPGA Trap Trig")
        n2715 = xnode "Read/Write Control"("FPGA VI Reference In"=w3471, "error in"=w3470, "FPGA Trap Trig"=w3469) -> ("FPGA VI Reference Out"=w3468:T20, "error out"=w3467:errorcluster)
        n2716 = xnode "Read/Write Control"("FPGA VI Reference In"=w3468, "error in"=w3467, "TTrig?"=w3469) -> ()  [unwired: 2 out]
        n2717 = local write "Initializing"(FALSE ("Initializing")) -> ()
        n2718 = local write "Triggered"(FALSE ("Triggered")) -> ()
        n2719 = local write "Waiting"(FALSE ("Waiting")) -> ()
      }
    }
    n2720 = Not(x=w3141) -> (.not. x?=w3154:bool)
    n2721 = And(x="Trap Trig. Fl.", y=w3154) -> (x .and. y?=w3151:bool)
    n2722 = local read "Tether"() -> (w3279:bool)
    n2723 = Or(x=w3151, y="Reinitialize") -> (x .or. y?=w3137:bool)
    n2724 = feedback #23(w3147) -> (w3152:string)
    n2725 = Select(t=w3147, s=w3151, f=w3152) -> (s? t:f=w3146:string)
    n2726 = Select(t=w3147, s="Reinitialize", f=w3146) -> (s? t:f=w3145:string)
    n2727 = feedback #24(0) -> (w3149:i32)
    n2728 = feedback #25(w3272) -> (w3271:dbl[])
    n2729 = Build Array (concatenate)(w3272, w3271) -> (w3105:dbl[])
    n2730 = case "For determining if there is a tether still" shown="True" w3279 {
      tunnel: w3278 -> [_ w3595]
      frame False {
      }
      frame True {
        n2731 = Greater?(x="Lost Tether Alarm Threshold (pN)", y=w3595) -> (0:w3593:bool)
        n2732 = case shown="True" w3593 {
          frame False {
          }
          frame True {
            w3596 = FALSE ("Value (Signaling)")
            n2733 = flat-sequence {
              frame #0 {
                # "stop only if saving"
                n2734 = local read "Saving..."() -> (w3608:bool)
                n2735 = And(x=w3608, y="TA Cancel Save?") -> (x .and. y?=w3607:bool)
                n2736 = local write "Stop Saving"(w3607) -> ()
              }
              frame #1 {
                n2737 = case shown="True" "TA Green Off?" {
                  frame False {
                  }
                  frame True {
                    w3611 = FALSE ("Fl. Triggered...")
                    n2738 = local write "Fl. Triggered..."(w3611) -> ()
                    n2739 = property on="Green Laser ON" class="Bool (strict)"("Val(Sgnl)"=w3611) -> ()  [unwired: 2 in, 2 out]
                  }
                }
              }
            }
            n2740 = local read "Time tether formed"() -> (w3602:timestamp)
            n2741 = Get Date/Time In Seconds() -> (seconds since 1Jan1904=w3603:timestamp)
            n2742 = Subtract(x=w3603, y=w3602) -> (x-y=w3601:dbl)
            n2743 = Number To Decimal String(number=w3601) -> (decimal integer string=w3598:string)  [unwired: 1 out]
            n2744 = local read "Messages"() -> (w3605:string)
            n2745 = call <vilib>:"Beep.vi"() -> ()  [unwired: 3 in, 9 out]
            n2746 = Concatenate Strings("Lost tether (" ("Message to add"), w3598, " s)." ("string")) -> (w3600:string)
            n2747 = local write "Tether"(FALSE ("Tether")) -> ()
            n2748 = call "Update messages.vi"("Message to add"=w3600, "Old message string"=w3605) -> ("New message string"=w3604:string)
            n2749 = local write "Messages"(w3604) -> ()
            n2750 = property on="Fl. Triggered..." class="Bool (strict)"("Val(Sgnl)"=w3596) -> ()  [unwired: 2 in, 2 out]
            n2751 = local write "Dip for Protein"(w3596) -> ()
            n2752 = property on="Trap Pos. FB ON" class="Bool (strict)"("Val(Sgnl)"=w3596) -> ()  [unwired: 2 in, 2 out]
            n2753 = property on="Trap Trig. Fl." class="Bool (strict)"("Val(Sgnl)"=w3596) -> ()  [unwired: 2 in, 2 out]
          }
        }
      }
    }
    n2754 = case "For triggering actions based on the trap position (e.g., turning the excitation laser on if trap under feedback moves so far)" shown="True" "Trap Trig. Fl." {
      tunnel: w3132 -> [_ w3484]
      tunnel: w3145 -> [_ w3483]
      tunnel: ["" ("t") w3482] -> w3153
      tunnel: w3137 -> [_ w3481]
      tunnel: [0 ("t") w3480] -> w3150
      tunnel: w3149 -> [_ w3479]
      tunnel: w3124 -> [_ w3478]
      tunnel: w3123 -> [_ w3477]
      frame False {
      }
      frame True {
        n2755 = case shown="\"Wait for trigger\"" w3483 {
          tunnel: w3484 -> [w3501 _ _ w3549]
          tunnel: [w3498 w3530 "" ("t") w3552] -> w3482
          tunnel: w3481 -> [_ _ _ w3540]
          tunnel: [w3497 w3527 0 ("t") w3541] -> w3480
          tunnel: w3479 -> [_ w3529 _ w3547]
          tunnel: w3478 -> [w3486 w3524 _ w3543]
          tunnel: w3477 -> [w3485 w3523 _ w3542]
          frame "Wait for trigger" {
            n2756 = local read "Trap Trig. (FPGA)"() -> (w3489:bool)
            n2757 = Subtract(x=w3501, y="Mean T1 Position\nto compare (nm)") -> (x-y=w3494:dbl[])
            n2758 = call <vilib>:"Std Deviation and Variance.vi"("X"=w3494) -> ("mean"=→"mean":dbl, "standard deviation"=→"standard\ndeviation":dbl)  [unwired: 1 in, 1 out]
            n2759 = Array Max & Min(array=w3494) -> (max value=→"max value":dbl, min value=→"min value":dbl)  [unwired: 2 out]
            n2760 = Greater?(x=w3494, y="Threshold (nm)") -> (0:w3504:bool[])
            n2761 = case shown="True" w3489 {
              tunnel: w3486 -> [_ w3510]
              tunnel: w3485 -> [_ w3509]
              tunnel: [FALSE ("TTrig?") w3508] -> w3492
              frame False {
              }
              frame True {
                n2762 = xnode "Read/Write Control"("FPGA VI Reference In"=w3510, "error in"=w3509) -> ("TTrig?"=w3508:bool)  [unwired: 2 out]
              }
            }
            n2763 = Or Array Elements(Boolean array=w3504) -> (logical OR=w3491:bool)
            n2764 = Select(t=w3492, s=w3489, f=w3491) -> (s? t:f=w3490:bool)
            n2765 = Not(x=w3489) -> (.not. x?=w3488:bool)
            n2766 = And(x=w3490, y=w3488) -> (x .and. y?=w3487:bool)
            n2767 = Select(t="Triggered", s=w3490, f="Wait for trigger") -> (s? t:f=w3498:string)
            n2768 = case shown="True" w3490 {
              tunnel: [0 0] -> w3497
              tunnel: w3486 -> [_ w3515]
              tunnel: w3485 -> [_ w3514]
              frame False {
                "Waiting" <- TRUE ("Waiting")
              }
              frame True {
                n2769 = xnode "Read/Write Control"("FPGA VI Reference In"=w3515, "error in"=w3514, "TTrig?"=FALSE) -> ()  [unwired: 2 out]
                n2770 = local read "Messages"() -> (w3518:string)
                n2771 = call <vilib>:"Beep.vi"() -> ()  [unwired: 12 in]
                n2772 = call "Update messages.vi"("Message to add"="Unwinding trigger.", "Old message string"=w3518) -> ("New message string"=w3519:string)
                n2773 = local write "Messages"(w3519) -> ()
                n2774 = local write "Waiting"(FALSE ("Waiting")) -> ()
                "Triggered" <- TRUE ("Triggered")
              }
            }
            n2775 = case "Only need to turn on laser if host triggered" shown="True" w3487 {
              frame False {
              }
              frame True {
                n2776 = property on="Green Laser ON" class="Bool (strict)"("Val(Sgnl)"=TRUE ("Value (Signaling)")) -> ()  [unwired: 2 in, 2 out]
              }
            }
          }
          frame "Triggered" {
            n2777 = local read "Trap Trig. (FPGA)"() -> (w3526:bool)
            n2778 = Increment(x=w3529) -> (x+1=w3527:i32)
            n2779 = Greater Or Equal?(x=w3527, y="Fl. ON time (n)") -> (x >= y?=w3525:bool)
            n2780 = Select(t="Wait for trigger", s=w3525, f="Triggered" ("t")) -> (s? t:f=w3530:string)
            n2781 = And(x=w3525, y=w3526) -> (x .and. y?=w3522:bool)
            n2782 = case shown="True" w3522 {
              tunnel: w3524 -> [_ w3534]
              tunnel: w3523 -> [_ w3533]
              frame False {
              }
              frame True {
                n2783 = xnode "Read/Write Control"("FPGA VI Reference In"=w3534, "error in"=w3533, "FPGA Trap Trig"=TRUE) -> ()  [unwired: 2 out]
              }
            }
            n2784 = case shown="True" w3525 {
              frame False {
              }
              frame True {
                w3536 = FALSE ("Value (Signaling)")
                n2785 = local write "Triggered"(w3536) -> ()
                n2786 = local write "Waiting"(TRUE ("Waiting")) -> ()
                n2787 = property on="Green Laser ON" class="Bool (strict)"("Val(Sgnl)"=w3536) -> ()  [unwired: 2 in, 2 out]
              }
            }
          }
          frame "Do nothing" {
          }
          frame "Initialize", Default {
            n2788 = Increment(x=w3547) -> (x+1=w3551:i32)
            n2789 = Select(t=1, s=w3540, f=w3551) -> (s? t:f=w3541:i32)
            n2790 = feedback #26(w3549) -> (w3555:dbl[])
            n2791 = Build Array (concatenate)(w3549, w3555) -> (w3548:dbl[])
            n2792 = Greater Or Equal?(x=w3541, y="Wait to get offset (n)") -> (x >= y?=w3544:bool)
            n2793 = Select(t=w3549, s=w3540, f=w3548) -> (s? t:f=w3550:dbl[])
            n2794 = feedback-in #26(w3550) -> ()
            n2795 = call-poly <vilib>:"Mean.vi"("X"=w3550) -> ("mean"=w3545:dbl)  [unwired: 1 out]
            n2796 = local write "Mean T1 Position\nto compare (nm)"(w3545) -> ()
            n2797 = case shown="True" w3540 {
              tunnel: w3543 -> [_ w3561]
              tunnel: w3542 -> [_ w3560]
              frame False {
              }
              frame True {
                w3557 = FALSE ("FPGA Trap Trig")
